vi "Main.vi"(8 "error in (no error)":errorcluster) -> (0 "error out":errorcluster)   [LabVIEW 2025]
uses:
  SubVIs/Controls/State_Machine_Ctrl.ctl
  SubVIs/Controls/TypeDef_FGV.ctl
  SubVIs/FGV/FGV_DO_Table.vi
  <vilib>/DAQmx/write.llb/DAQmx Write (Digital 1D U32 1Chan NSamp).vi
  <vilib>/DAQmx/write.llb/DAQmx Write (Analog 1D Wfm NChan NSamp).vi
panel:
  out "Dimension":i32
  out "DO WF":waveform(dbl)(graph)
  in  "Wait_mirror_s":dbl=0.5
  in  "Type of pattern":T1(ring)
  in  "sample mode":i32(ring)=10123 items=["Échantillons finis"=10178, "Échantillons continus"=10123, "Point par point avec cadencement matériel"=12522]
  out "AO WF":waveform(dbl)[](graph)
  in  "Readout time (s)":dbl=0.5
  in  "Exposure time (s)":dbl=0.1
  in  "Start":bool
  in  "Stop":bool
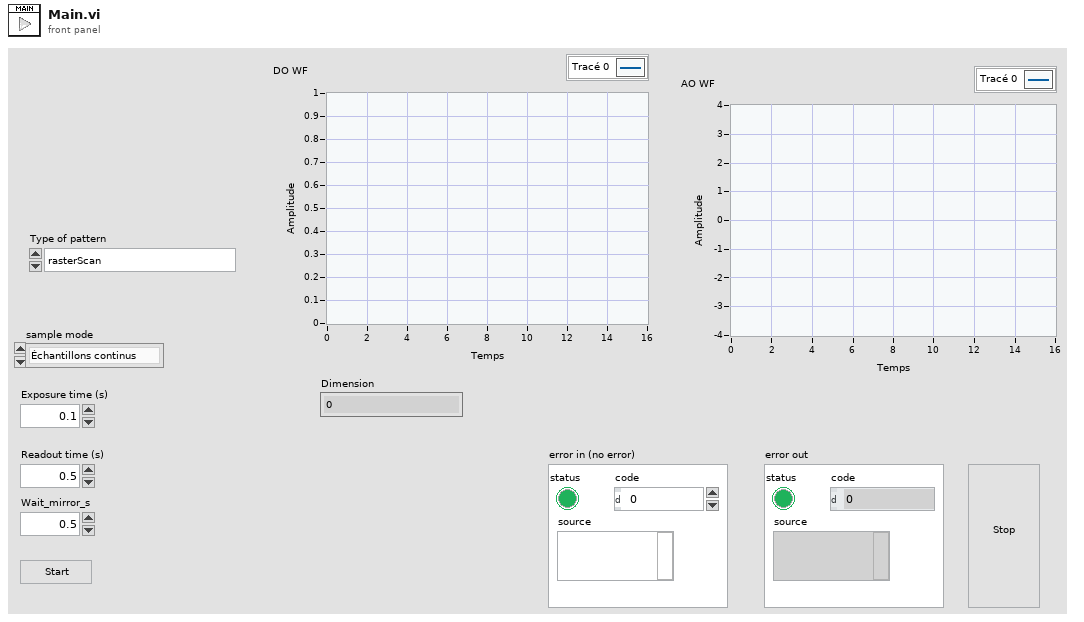
[diagram p1: front panel]
types:
  T1 = enum16{"rasterScan", "snakeMovement", "circularScan", "circularTIR", "spiralScan"}
  T2 = typedef "State_Machine_Ctrl.ctl" = enum16{"Initialize", "Wait for Event", "Setup_DAQ", "Create WF", "Generate WF", "Stop"}
  T3 = typedef "TypeDef_FGV.ctl" = enum16{"Initialize", "Write", "Read"}
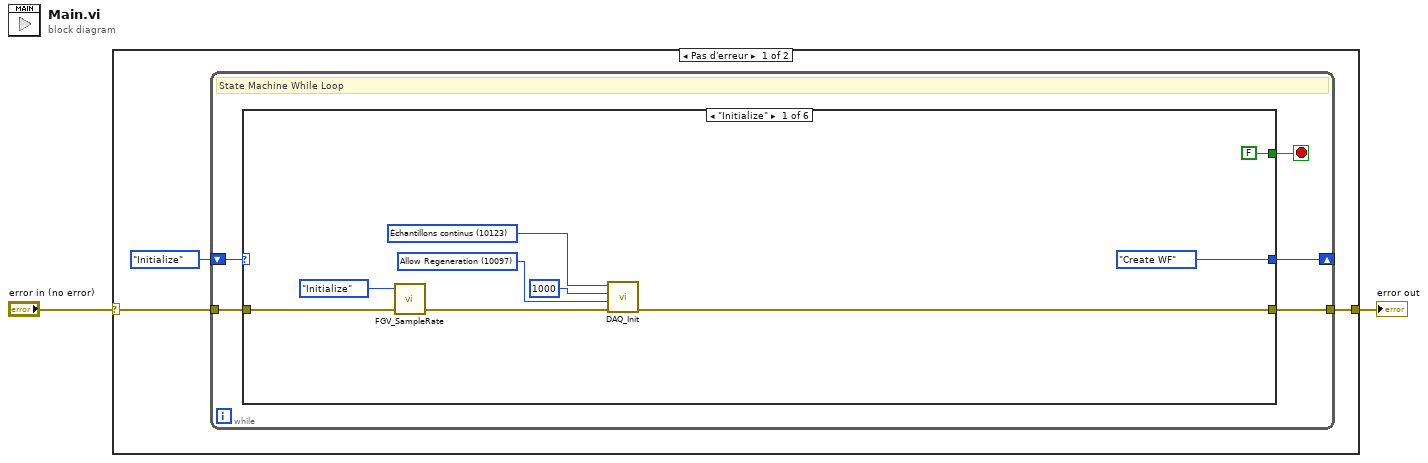
[diagram p0: block diagram]
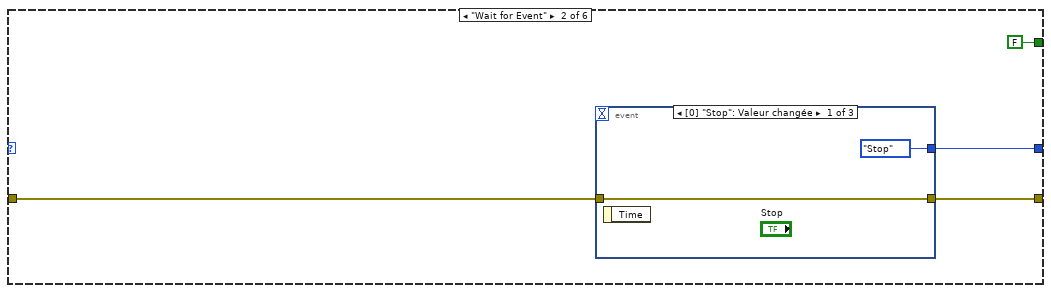
[diagram p2: hidden frame]
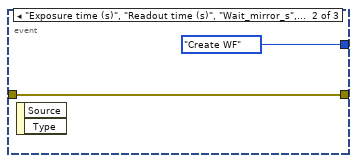
[diagram p3: hidden frame]
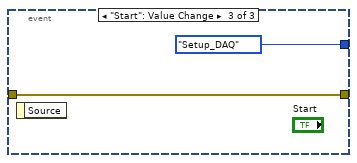
[diagram p4: hidden frame]
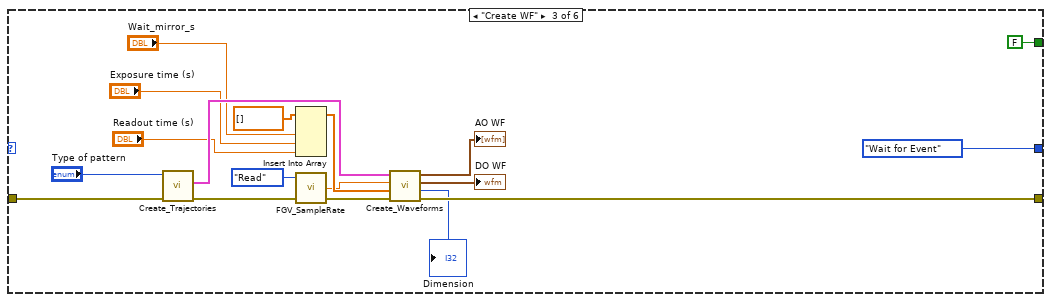
[diagram p5: hidden frame]
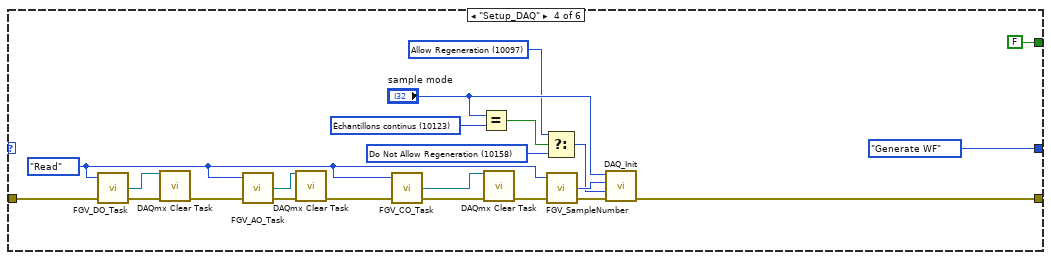
[diagram p6: hidden frame]
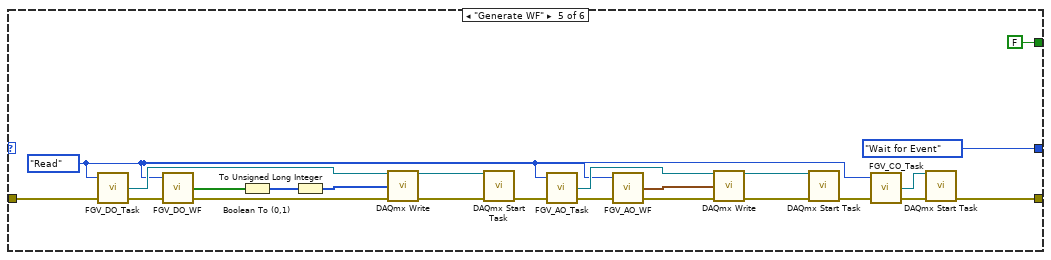
[diagram p7: hidden frame]
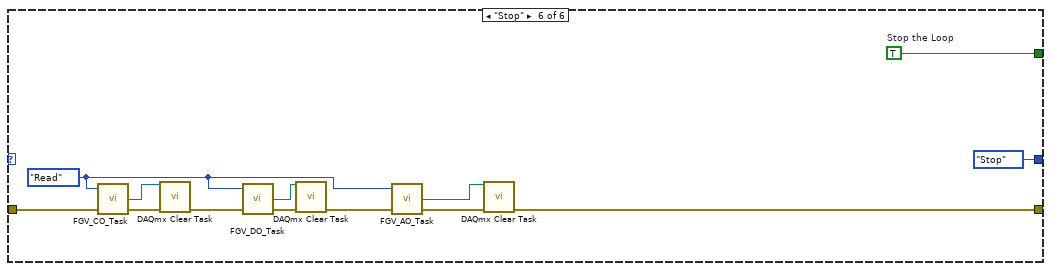
[diagram p8: hidden frame]
diagram:
  n1 = case shown="Pas d'erreur" "error in (no error)" {
    selector: "error in (no error)" -> [w4 w106]
    tunnel: [w3 w106] -> w2
    frame No Error {
      n2 = while {
        shift-right: [w9] -> _
        shift-left: State_Machine_Ctrl."Initialize" ("Initial State") -> [w10]
        tunnel: w4 -> [w7]
        tunnel: [w6] -> w3
        stop <- w8 stop-if-true
        # "State Machine While Loop"
        n3 = case "State Machine Case Structure" shown="\"Initialize\"" w10 {
          tunnel: [State_Machine_Ctrl."Create WF" ("Initial State") w23 State_Machine_Ctrl."Wait for Event" ("Initial State") State_Machine_Ctrl."Generate WF" ("Initial State") State_Machine_Ctrl."Wait for Event" ("Initial State") State_Machine_Ctrl."Stop" ("Initial State")] -> w9
          tunnel: [FALSE ("Stop the Loop") FALSE ("Stop the Loop") FALSE ("Stop the Loop") FALSE ("Stop the Loop") FALSE ("Stop the Loop") w105] -> w8
          tunnel: w7 -> [w16 w21 w44 w67 w89 w102]
          tunnel: [w12 w20 w31 w54 w73 w98] -> w6
          frame "Initialize" {
            w11 = 10097 items=["Allow Regeneration"=10097, "Do Not Allow Regeneration"=10158] ("RegenMode")
            w15 = 10123 items=["Échantillons finis"=10178, "Échantillons continus"=10123, "Point par point avec cadencement matériel"=12522] ("sample mode")
            # "Initialize - In this example, the only initialization required is to specify that the next state for the state machine is \"Wait for Event\"."
            n4 = call "FGV_SampleRate.vi"("error in"=w16, "Action"=TypeDef_FGV."Initialize") -> ("error out"=w13:errorcluster)  [unwired: 2 in, 1 out]
            n5 = call "DAQ_Init.vi"("error in"=w13, "RegenMode"=w11, "samples per channel"=1000, "sample mode"=w15) -> ("error out"=w12:errorcluster)  [unwired: 7 in]
          }
          frame "Wait for Event" {
            # "Wait for Event - An Event Structure is used to monitor the user interface for events. In each frame of the Event Structure, the next state of the state machine is specified based on which button was pressed."
            n6 = event shown="[0] \"Stop\": Valeur changée" {
              selector: _ -> [_ _ _]
              dyn-events: _ -> [_ _ _]
              timeout: _ -> [_ _ _]
              tunnel: [State_Machine_Ctrl."Stop" ("Initial State") State_Machine_Ctrl."Create WF" ("Initial State") State_Machine_Ctrl."Setup_DAQ" ("Initial State")] -> w23
              tunnel: w21 -> [w24 w27 w28]
              tunnel: [w24 w27 w28] -> w20
              event "Stop": Value Change {
                n7 = event-data() -> ()  [unwired: 1 in, 1 out]
              }
              event "Exposure time (s)", "Readout time (s)", "Wait_mirror_s", "Type of pattern", "sample mode": Value Change {
                n8 = event-data() -> ()  [unwired: 1 in, 2 out]
              }
              event "Start": Value Change {
                n9 = event-data() -> ()  [unwired: 1 in, 1 out]
              }
            }
          }
          frame "Create WF" {
            n10 = call "Create_Trajectories.vi"("error in"=w44, "Type of pattern"="Type of pattern") -> ("error out"=w41:errorcluster, "Trajectories"=w43:cluster{dbl[], dbl[]})  [unwired: 7 in, 1 out]
            n11 = Insert Into Array(array=dbl[] [] ("tableau"), new element #1="Wait_mirror_s", new element #2="Exposure time (s)", new element #3="Readout time (s)") -> (w42:dbl[])  [unwired: 1 in]
            n12 = call "FGV_SampleRate.vi"("error in"=w41, "Action"=TypeDef_FGV."Read") -> ("error out"=w40:errorcluster, "CO task"=w34:dbl)  [unwired: 2 in]
            n13 = call "Create_Waveforms.vi"("error in"=w40, "Timings (sleep, expo, readout) _s"=w42, "sample_rate_Hz"=w34, "Trajectories"=w43) -> ("error out"=w31:errorcluster, "Dimension"=→"Dimension":i32, "DO WF"=→"DO WF":waveform(dbl), "AO WF"=→"AO WF":waveform(dbl)[])  [unwired: 4 in]
          }
          frame "Setup_DAQ" {
            w49 = 10158 items=["Allow Regeneration"=10097, "Do Not Allow Regeneration"=10158] ("RegenMode")
            w50 = 10097 items=["Allow Regeneration"=10097, "Do Not Allow Regeneration"=10158] ("RegenMode")
            w53 = 10123 items=["Échantillons finis"=10178, "Échantillons continus"=10123, "Point par point avec cadencement matériel"=12522] ("sample mode 2")
            w57 = TypeDef_FGV."Read" ("Action")
            n14 = call "FGV_DO_Task.vi"("error in"=w67, "Action"=w57) -> ("error out"=w66:errorcluster, "CO task"=w65:refnum<k21>)  [unwired: 2 in]
            n15 = call <vilib>:"DAQmx Clear Task.vi"("task in"=w65, "error in"=w66) -> ("error out"=w64:errorcluster)  [unwired: 13 in]
            n16 = call "FGV_AO_Task.vi"("error in"=w64, "Action"=w57) -> ("error out"=w63:errorcluster, "CO task"=w62:refnum<k21>)  [unwired: 2 in]
            n17 = call <vilib>:"DAQmx Clear Task.vi"("task in"=w62, "error in"=w63) -> ("error out"=w61:errorcluster)  [unwired: 13 in]
            n18 = call "FGV_CO_Task.vi"("error in"=w61, "Action"=w57) -> ("error out"=w60:errorcluster, "CO task"=w59:refnum<k21>)  [unwired: 2 in]
            n19 = Equal?(x="sample mode", y=w53) -> (x = y?=w52:bool)
            n20 = call <vilib>:"DAQmx Clear Task.vi"("task in"=w59, "error in"=w60) -> ("error out"=w58:errorcluster)  [unwired: 13 in]
            n21 = Select(t=w50, s=w52, f=w49) -> (s? t:f=w48:i32)
            n22 = call "FGV_SampleNumber.vi"("error in"=w58, "Action"=w57) -> ("error out"=w55:errorcluster, "Sample number"=w56:u32)  [unwired: 2 in]
            n23 = call "DAQ_Init.vi"("error in"=w55, "RegenMode"=w48, "samples per channel"=w56, "sample mode"="sample mode") -> ("error out"=w54:errorcluster)  [unwired: 7 in]
          }
          frame "Generate WF" {
            w75 = TypeDef_FGV."Read" ("Action")
            n24 = call "FGV_DO_Task.vi"("error in"=w89, "Action"=w75) -> ("error out"=w86:errorcluster, "CO task"=w88:refnum<k21>)  [unwired: 2 in]
            n25 = call "FGV_DO_WF.vi"("error in"=w86, "Action"=w75) -> ("error out"=w87:errorcluster, "DO table"=w72:bool[])  [unwired: 2 in]
            n26 = Boolean To (0,1)(Boolean=w72) -> (0, 1=w70:i16[])
            n27 = To Unsigned Long Integer(number=w70) -> (unsigned 32bit integer=w71:u32[])
            n28 = call-poly <vilib>:"DAQmx Write.vi"("task/channels in"=w88, "data"=w71, "error in"=w87) -> ("task out"=w84:refnum<k21>, "error out"=w83:errorcluster)  [unwired: 10 in, 1 out]
            n29 = call <vilib>:"DAQmx Start Task.vi"("task/channels in"=w84, "error in"=w83) -> ("error out"=w82:errorcluster)  [unwired: 12 in, 1 out]
            n30 = call "FGV_AO_Task.vi"("error in"=w82, "Action"=w75) -> ("error out"=w79:errorcluster, "CO task"=w85:refnum<k21>)  [unwired: 2 in]
            n31 = call "FGV_AO_WF.vi"("error in 2"=w79, "Action 2"=w75) -> ("error out 2"=w78:errorcluster, "AO WF 2"=w77:waveform(dbl)[])  [unwired: 2 in]
            n32 = call-poly <vilib>:"DAQmx Write.vi"("task/channels in"=w85, "data"=w77, "error in"=w78) -> ("task out"=w80:refnum<k21>, "error out"=w81:errorcluster)  [unwired: 10 in, 1 out]
            n33 = call <vilib>:"DAQmx Start Task.vi"("task/channels in"=w80, "error in"=w81) -> ("error out"=w74:errorcluster)  [unwired: 12 in, 1 out]
            n34 = call "FGV_CO_Task.vi"("error in"=w74, "Action"=w75) -> ("error out"=w76:errorcluster, "CO task"=w90:refnum<k21>)  [unwired: 2 in]
            n35 = call <vilib>:"DAQmx Start Task.vi"("task/channels in"=w90, "error in"=w76) -> ("error out"=w73:errorcluster)  [unwired: 12 in, 1 out]
          }
          frame "Stop" {
            w103 = TypeDef_FGV."Read" ("Action")
            w105 = TRUE  # Stop the Loop
            # "Stop - Stop the VI. This is the only state that specifies a TRUE value for the loop conditional terminal."
            n36 = call "FGV_CO_Task.vi"("error in"=w102, "Action"=w103) -> ("error out"=w100:errorcluster, "CO task"=w101:refnum<k21>)  [unwired: 2 in]
            n37 = call <vilib>:"DAQmx Clear Task.vi"("task in"=w101, "error in"=w100) -> ("error out"=w99:errorcluster)  [unwired: 13 in]
            n38 = call "FGV_DO_Task.vi"("error in"=w99, "Action"=w103) -> ("error out"=w95:errorcluster, "CO task"=w94:refnum<k21>)  [unwired: 2 in]
            n39 = call <vilib>:"DAQmx Clear Task.vi"("task in"=w94, "error in"=w95) -> ("error out"=w96:errorcluster)  [unwired: 13 in]
            n40 = call "FGV_AO_Task.vi"("error in"=w96, "Action"=w103) -> ("error out"=w97:errorcluster, "CO task"=w93:refnum<k21>)  [unwired: 2 in]
            n41 = call <vilib>:"DAQmx Clear Task.vi"("task in"=w93, "error in"=w97) -> ("error out"=w98:errorcluster)  [unwired: 13 in]
          }
        }
      }
    }
    frame Error {
    }
  }
  "error out" <- w2
